vi "Constructor_SQLiteLogHandle_Inject.vi"(7 "TableName (event_log)":string="event_log", 8 "error in (no error)":errorcluster, 11 "Connection in":refnum<class "Connection.lvclass">) -> (0 "error out":errorcluster, 3 "SQLiteLogHandle out":refnum<class "SQLiteLogHandle.lvclass">)   [LabVIEW 2024, in "SQLiteLogHandle.lvclass"]
uses:
  SQLiteLogHandle.lvclass
  <vilib>/drjdpowell/SQLite Library/SQL Connection/Connection.lvclass
  SQLiteLogHandle.lvclass/SQLiteLogHandle.ctl
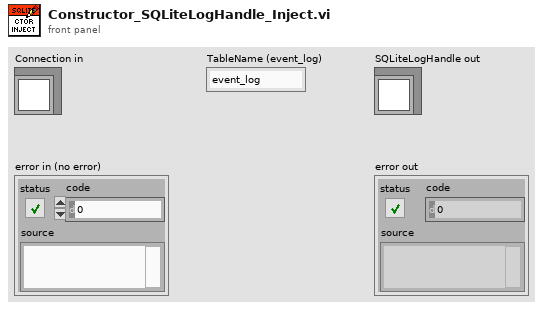
[diagram p1: front panel]
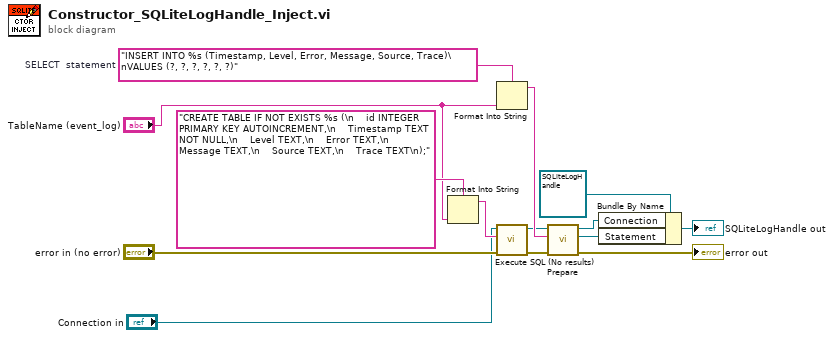
[diagram p0: block diagram]
diagram:
  w13 = "INSERT INTO %s (Timestamp, Level, Error, Message, Source, Trace)\nVALUES (?, ?, ?, ?, ?, ?)"  # SELECT  statement
  n1 = Format Into String(format string="CREATE TABLE IF NOT EXISTS %s (\n    id INTEGER PRIMARY KEY AUTOINCREMENT,\n    Timestamp TEXT NOT NULL,\n    Level TEXT,\n    Error TEXT,\n    Message TEXT,\n    Source TEXT,\n    Trace TEXT\n);", "TableName (event_log)") -> (resulting string=w7:string)  [unwired: 2 in, 1 out]
  n2 = Format Into String(format string=w13, "TableName (event_log)") -> (resulting string=w14:string)  [unwired: 2 in, 1 out]
  n3 = call <vilib>:"Execute SQL (No results).vi"("error in (no error)"="error in (no error)", "SQL"=w7, "SQLite Connection in"="Connection in") -> ("error out"=w5:errorcluster, "SQLite Connection"=w4:refnum<class "Connection.lvclass">)  [unwired: 7 in]
  n4 = call <vilib>:"Prepare.vi"("error in (no error)"=w5, "SQL"=w14, "SQLite Connection in"=w4) -> ("error out"=→"error out":errorcluster, "SQL Statement"=w12:refnum<class "SQL Statement.lvclass">, "SQLite Connection"=w2:refnum<class "Connection.lvclass">)  [unwired: 4 in, 2 out]
  n5 = Bundle By Name(cluster=refnum<class "SQLiteLogHandle.lvclass"> refnum ("SQLiteLogHandle in"), "Connection"=w2, "Statement"=w12) -> (→"SQLiteLogHandle out":refnum<class "SQLiteLogHandle.lvclass">)
